vi "Video feed info class VI - change video state.vi"(8 "error in (no error)":errorcluster, 10 "video state":T1(ring), 11 "Video feed info in":refnum<class "Video feed info.lvclass">) -> (0 "error out":errorcluster, 3 "Video feed info out":refnum<class "Video feed info.lvclass">)   [LabVIEW 2010, in "Video feed info.lvclass"]
uses:
  Video feed info.lvclass
  Video feed info.lvclass/Video feed info.ctl
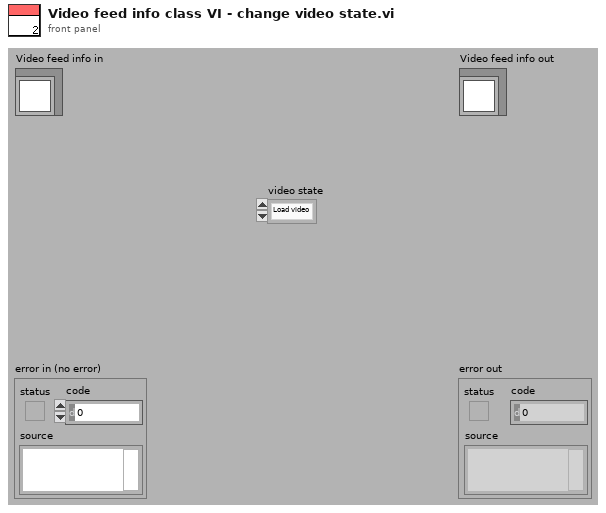
[diagram p1: front panel]
types:
  T1 = enum16{"Load video", "Idle", "Play", "Rewind", "Forward"}
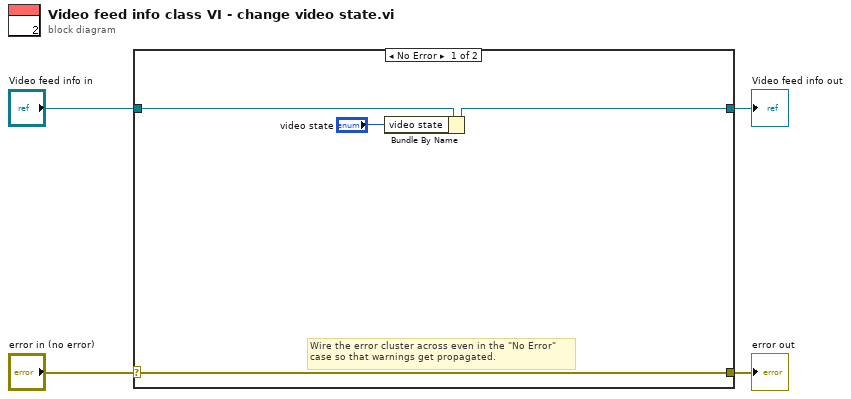
[diagram p0: block diagram]
diagram:
  n1 = case shown="No Error" "error in (no error)" {
    selector: "error in (no error)" -> [w7 w10]
    tunnel: [w7 w10] -> w3
    tunnel: [w6 w9] -> w1
    tunnel: "Video feed info in" -> [w8 w9]
    frame No Error {
      # "Wire the error cluster across even in the \"No Error\"\ncase so that warnings get propagated."
      n2 = Bundle By Name(cluster=w8, "video state"="video state") -> (w6:refnum<class "Video feed info.lvclass">)
    }
    frame Error {
    }
  }
  "error out" <- w3
  "Video feed info out" <- w1
